vi "Ex1_Arrays.vi"() -> ()   [LabVIEW 2024]
panel:
  out "Element":dbl
  out "size(s)":i32
  in  "Array 3":bool[](array[boolean])
  out "Array 2":dbl[](array[numeric])
  in  "Array":dbl[](array[numeric])
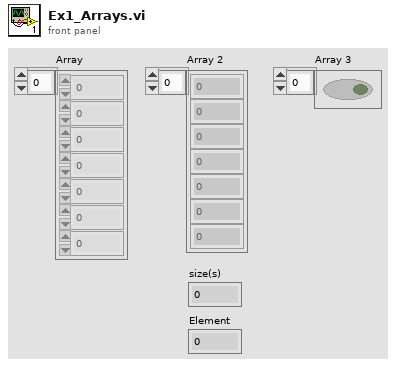
[diagram p1: front panel]
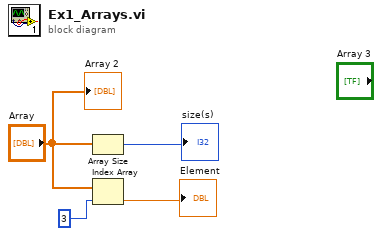
[diagram p0: block diagram]
diagram:
  n1 = Array Size(array="Array") -> (size(s)=→"size(s)":i32)
  n2 = Index Array(array="Array", index=3) -> (element=→"Element":dbl)
  "Array 2" <- "Array"
